vi "SWERVE_TRAJECTORY_ODOM_EXECUTE.vi"(6 "Initial Pose":T2={"TRANSLATION"={"X"=0.0, "Y"=0.0}, "ROTATION"={"VALUE"=0.0, "COS"=1.0, "SIN"=0.0}} {"ROTATION"."SIN" format="%13.4f"; "ROTATION"."COS" format="%13.4f"; "ROTATION"."VALUE" format="%13.4f"; "TRANSLATION"."Y" format="%14.3f"; "TRANSLATION"."X" format="%14.3f"}, 8 "Init":bool, 9 "ROTATION":T4 {"SIN" format="%13.4f"; "COS" format="%13.4f"; "VALUE" format="%13.4f"}, 10 "Swerve Module Positions":T5[](array[typedef]) {"Angle"."SIN" format="%13.4f"; "Angle"."COS" format="%13.4f"; "Angle"."VALUE" format="%13.4f"}, 11 "out SWERVE_DRIVE_KINEMATICS":T6 {"SavedModuleStates"."Angle"."SIN" format="%13.4f"; "SavedModuleStates"."Angle"."COS" format="%13.4f"; "SavedModuleStates"."Angle"."VALUE" format="%13.4f"; "PrevCoR"."Y" format="%14.3f"; "PrevCoR"."X" format="%14.3f"; "Modules"."Y" format="%14.3f"; "Modules"."X" format="%14.3f"}) -> (0 "Error":bool, 3 "robot POSE":T2 {"ROTATION"."SIN" format="%13.4f"; "ROTATION"."COS" format="%13.4f"; "ROTATION"."VALUE" format="%13.4f"; "TRANSLATION"."Y" format="%14.3f"; "TRANSLATION"."X" format="%14.3f"}, 4 "out SWERVE_DRIVE_ODOMETRY":T1={"POSE"={"TRANSLATION"={"X"=0.0, "Y"=0.0}, "ROTATION"={"VALUE"=0.0, "COS"=1.0, "SIN"=0.0}}, "GyroOffset"={"VALUE"=0.0, "COS"=1.0, "SIN"=0.0}, "PreviousAngle"={"VALUE"=0.0, "COS"=1.0, "SIN"=0.0}, "PrevModulePositions"=[], "NumModules"=0} {"PrevModulePositions"."Angle"."SIN" format="%13.4f"; "PrevModulePositions"."Angle"."COS" format="%13.4f"; "PrevModulePositions"."Angle"."VALUE" format="%13.4f"; "PreviousAngle"."SIN" format="%13.4f"; "PreviousAngle"."COS" format="%13.4f"; "PreviousAngle"."VALUE" format="%13.4f"; "GyroOffset"."SIN" format="%13.4f"; "GyroOffset"."COS" format="%13.4f"; "GyroOffset"."VALUE" format="%13.4f"; "POSE"."ROTATION"."SIN" format="%13.4f"; "POSE"."ROTATION"."COS" format="%13.4f"; "POSE"."ROTATION"."VALUE" format="%13.4f"; "POSE"."TRANSLATION"."Y" format="%14.3f"; "POSE"."TRANSLATION"."X" format="%14.3f"})   [LabVIEW 2019]
uses:
  <vilib>/Rock Robotics/WPI/ThirdParty/JAS_Junk/TrajLib/TypeDef/SWERVE_DRIVE_MODULE_POSITION.ctl
  <vilib>/Rock Robotics/WPI/ThirdParty/JAS_Junk/TrajLib/TypeDef/ROTATION2D.ctl
  <vilib>/Rock Robotics/WPI/ThirdParty/JAS_Junk/TrajLib/TypeDef/SWERVE_DRIVE_KINEMATICS.ctl
  <vilib>/Analysis/Matrix/Datatypes/RealMatrix.ctl
  <vilib>/Rock Robotics/WPI/ThirdParty/JAS_Junk/TrajLib/TypeDef/TRANSLATION2D.ctl
  <vilib>/Rock Robotics/WPI/ThirdParty/JAS_Junk/TrajLib/TypeDef/SWERVE_DRIVE_MODULE_STATE.ctl
  <vilib>/Rock Robotics/WPI/ThirdParty/JAS_Junk/TrajLib/TypeDef/POSE2D.ctl
  <vilib>/Rock Robotics/WPI/ThirdParty/JAS_Junk/TrajLib/Rotation2d_CreateAngle.vi
  <vilib>/Rock Robotics/WPI/ThirdParty/JAS_Junk/TrajLib/Translation2d_Create.vi
  <vilib>/Rock Robotics/WPI/ThirdParty/JAS_Junk/TrajLib/Pose2d_getRotation.vi
  <vilib>/Rock Robotics/WPI/ThirdParty/JAS_Junk/TrajLib/Rotation2d_Minus.vi
  <vilib>/Rock Robotics/WPI/ThirdParty/JAS_Junk/TrajLib/Rotation2d_UnaryMinus.vi
  <vilib>/Rock Robotics/WPI/ThirdParty/JAS_Junk/TrajLib/Rotation2d_RotateBy.vi
  <vilib>/Rock Robotics/WPI/ThirdParty/JAS_Junk/TrajLib/Rotation2d_CreateXY.vi
  <vilib>/Rock Robotics/WPI/ThirdParty/JAS_Junk/TrajLib/Util_CalcDist.vi
  <vilib>/Rock Robotics/WPI/ThirdParty/JAS_Junk/TrajLib/Trajectory_Library.lvlib
  <vilib>/Analysis/Matrix/NI_Matrix.lvlib
  <vilib>/Rock Robotics/WPI/ThirdParty/JAS_Junk/TrajLib/TypeDef/SWERVE_DRIVE_ODOMETRY.ctl
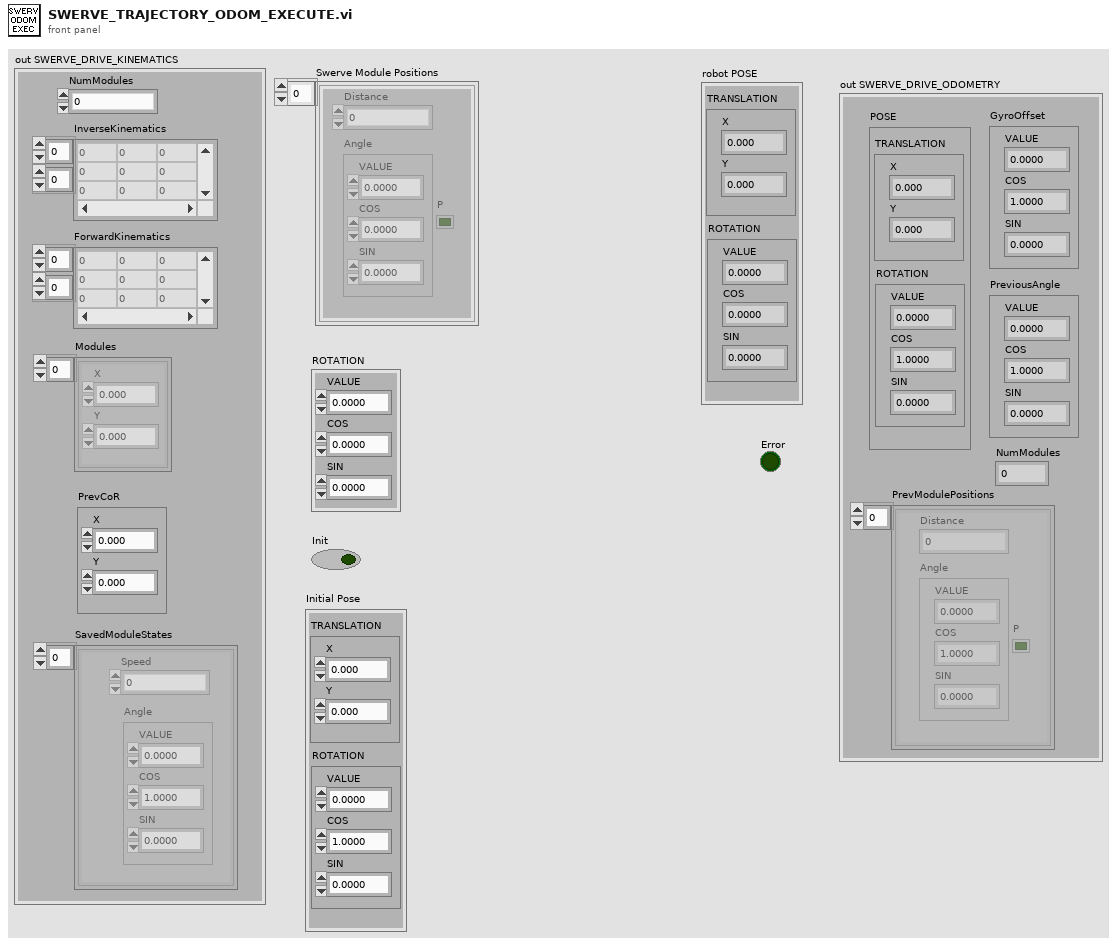
[diagram p1: front panel]
types:
  T1 = typedef "Trajectory_Library.lvlib/SWERVE_DRIVE_ODOMETRY.ctl" = cluster{"POSE":T2, "GyroOffset":T4, "PreviousAngle":T4, "PrevModulePositions":T5[], "NumModules":i32}
  T2 = typedef "Trajectory_Library.lvlib/POSE2D.ctl" = cluster{"TRANSLATION":T3, "ROTATION":T4}
  T3 = typedef "Trajectory_Library.lvlib/TRANSLATION2D.ctl" = cluster{"X":dbl, "Y":dbl}
  T4 = typedef "Trajectory_Library.lvlib/ROTATION2D.ctl" = cluster{"VALUE":dbl, "COS":dbl, "SIN":dbl}
  T5 = typedef "Trajectory_Library.lvlib/SWERVE_DRIVE_MODULE_POSITION.ctl" = cluster{"Distance":dbl, "Angle":T4, "P":bool}
  T6 = typedef "Trajectory_Library.lvlib/SWERVE_DRIVE_KINEMATICS.ctl" = cluster{"NumModules":i32, "InverseKinematics":T7, "ForwardKinematics":T7, "Modules":T3[], "PrevCoR":T3, "SavedModuleStates":T8[]}
  T7 = typedef "NI_Matrix.lvlib/RealMatrix.ctl" = dbl[][]
  T8 = typedef "Trajectory_Library.lvlib/SWERVE_DRIVE_MODULE_STATE.ctl" = cluster{"Speed":dbl, "Angle":T4}
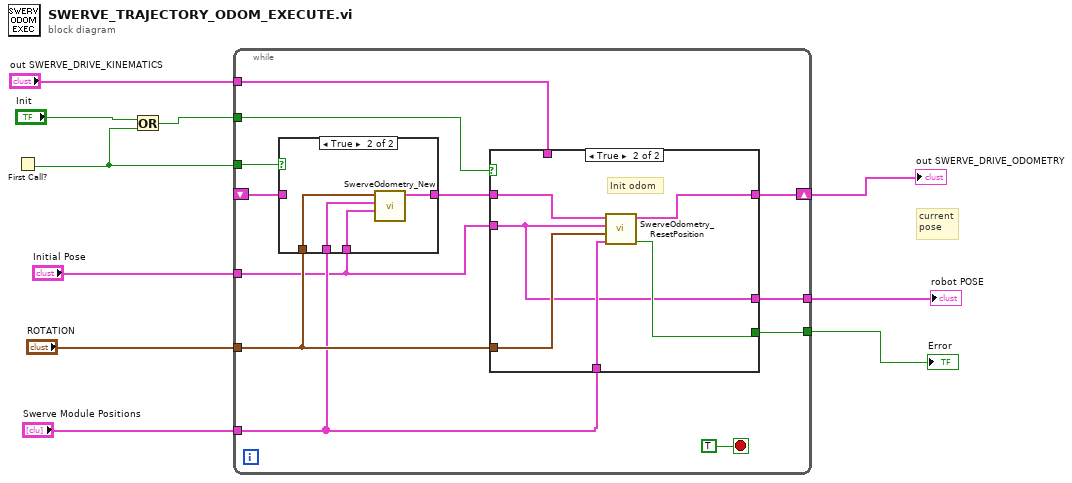
[diagram p0: block diagram]
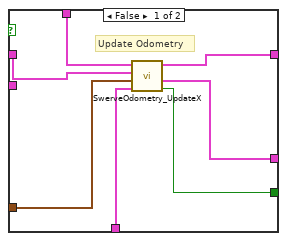
[diagram p3: hidden frame]
diagram:
  # "current\npose"
  n1 = First Call?() -> (First Call?: T/F=w2:bool)
  n2 = Or(x="Init", y=w2) -> (x .or. y?=w4:bool)
  n3 = while {
    tunnel: "Swerve Module Positions" -> [w14]
    tunnel: "ROTATION" -> [w15]
    tunnel: "out SWERVE_DRIVE_KINEMATICS" -> [w20]
    tunnel: [w18] -> w7
    tunnel: w4 -> [w22]
    shift-right: [w19] -> w1
    shift-left: _ -> [w11]
    tunnel: [w17] -> w6
    tunnel: "Initial Pose" -> [w13]
    tunnel: w2 -> [w16]
    stop <- TRUE stop-if-true
    n4 = case shown="True" w16 {
      tunnel: w15 -> [_ w27]
      tunnel: w14 -> [_ w26]
      tunnel: w13 -> [_ w25]
      tunnel: [w23 w24] -> w12
      tunnel: w11 -> [w23 _]
      frame False {
      }
      frame True {
        n5 = call <vilib>:"SwerveOdometry_New.vi"("InitialPose"=w25, "Module Positions"=w26, "gyroAngle"=w27) -> ("SWERVE_DRIVE_ODOMETRY"=w24:T1)  [unwired: 8 in]
      }
    }
    n6 = case shown="True" w22 {
      tunnel: w12 -> [w31 w40]
      tunnel: w15 -> [w30 w39]
      tunnel: w14 -> [w32 w38]
      tunnel: w20 -> [w34 _]
      tunnel: [w33 w37] -> w19
      tunnel: [w29 w35] -> w18
      tunnel: [w28 w36] -> w17
      tunnel: w13 -> [_ w35]
      frame False {
        # "Update Odometry"
        n7 = call <vilib>:"SwerveOdometry_UpdateX.vi"("module Positions"=w32, "gyroAngle"=w30, "in SWERVE_DRIVE_ODOMETRY"=w31, "SWERVE_DRIVE_KINEMATICS"=w34) -> ("Error"=w28:bool, "robot POSE"=w29:T2, "out SWERVE_DRIVE_ODOMETRY"=w33:T1)  [unwired: 5 in]
      }
      frame True {
        # "Init odom"
        n8 = call <vilib>:"SwerveOdometry_ResetPosition.vi"("Module Positions"=w38, "gyroAngle"=w39, "Pose"=w35, "in SWERVE_DRIVE_ODOMETRY"=w40) -> ("Error"=w36:bool, "out SWERVE_DRIVE_ODOMETRY"=w37:T1)  [unwired: 6 in]
      }
    }
  }
  "robot POSE" <- w7
  "Error" <- w6
  "out SWERVE_DRIVE_ODOMETRY" <- w1
